vi "DT3120_GetFrameSize.vi"(8 "error in (no error)":errorcluster, 10 "Source":u16, 11 "DevId":i32) -> (0 "error out":errorcluster, 2 "Frame Size":T1, 3 "DevId (dup)":i32)   [LabVIEW 2013]
uses:
  olfg32.dll
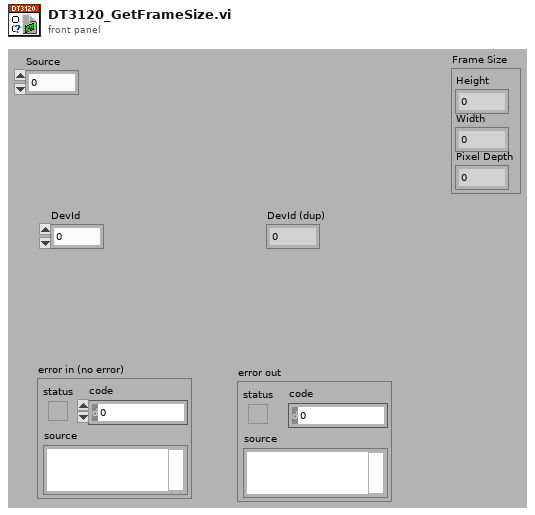
[diagram p1: front panel]
types:
  T1 = cluster{"Height":u32, "Width":u32, "Pixel Depth":u32}
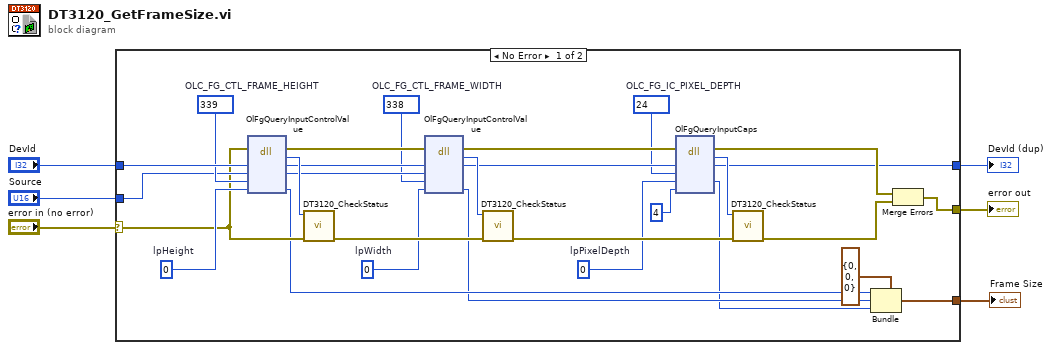
[diagram p0: block diagram]
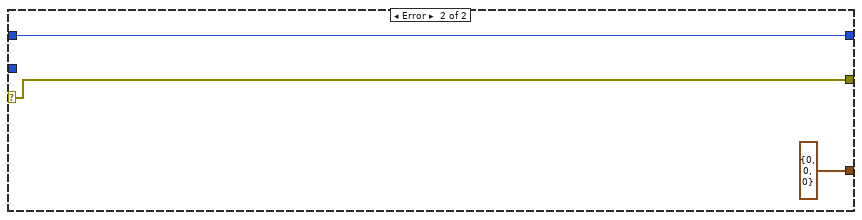
[diagram p2: hidden frame]
diagram:
  n1 = case shown="No Error" "error in (no error)" {
    selector: "error in (no error)" -> [w16 w38]
    tunnel: "DevId" -> [w34 w37]
    tunnel: "Source" -> [w27 _]
    tunnel: [w18 w38] -> w4
    tunnel: [w17 w37] -> w3
    tunnel: [w8 T1 {"Height"=0, "Width"=0, "Pixel Depth"=0} ("Frame Size")] -> w1
    frame No Error {
      w12 = u32 0  # lpPixelDepth
      w14 = 24  # OLC_FG_IC_PIXEL_DEPTH
      w15 = 338  # OLC_FG_CTL_FRAME_WIDTH
      w28 = u32 0  # lpWidth
      w32 = u32 0  # lpHeight
      w33 = 339  # OLC_FG_CTL_FRAME_HEIGHT
      n2 = dll-call lib="C:/Users/dhaehnel/Documents/Workspace/Labview_Workspace/labviewlib/MT Scan/SubVIs/olfg32.dll" fn="OlFgQueryInputControlValue"(error in=w16, "DevId"=w34, "Source"=w27, "Key"=w33, "lpValue"=w32) -> (error out=w31:errorcluster, "Status"=w35:u32, "DevId"=w25:i32, "Source"=w26:u16, "lpValue"=w11:u32)  [unwired: 3 in, 1 out]
      n3 = call "DT3120_CheckStatus.vi"("error in"=w16, "Status"=w35) -> ("error out"=w30:errorcluster)  [unwired: 9 out]
      n4 = dll-call lib="C:/Users/dhaehnel/Documents/Workspace/Labview_Workspace/labviewlib/MT Scan/SubVIs/olfg32.dll" fn="OlFgQueryInputControlValue"(error in=w31, "DevId"=w25, "Source"=w26, "Key"=w15, "lpValue"=w28) -> (error out=w23:errorcluster, "Status"=w29:u32, "DevId"=w24:i32, "lpValue"=w10:u32)  [unwired: 4 in, 1 out]
      n5 = call "DT3120_CheckStatus.vi"("error in"=w30, "Status"=w29) -> ("error out"=w21:errorcluster)  [unwired: 9 out]
      n6 = dll-call lib="C:/Users/dhaehnel/Documents/Workspace/Labview_Workspace/labviewlib/MT Scan/SubVIs/olfg32.dll" fn="OlFgQueryInputCaps"(error in=w23, "DevId"=w24, "Key"=w14, "lpData"=w12, "DataSize"=u32 4) -> (error out=w20:errorcluster, "Status"=w22:u32, "DevId"=w17:i32, "lpData"=w9:u32)  [unwired: 4 in, 1 out]
      n7 = call "DT3120_CheckStatus.vi"("error in"=w21, "Status"=w22) -> ("error out"=w19:errorcluster)  [unwired: 9 out]
      n8 = Bundle(cluster=T1 {"Height"=0, "Width"=0, "Pixel Depth"=0} ("Frame Size"), "Height"=w11, "Width"=w10, "Pixel Depth"=w9) -> (w8:T1)
      n9 = Merge Errors(w20, w19) -> (w18:errorcluster)
    }
    frame Error {
    }
  }
  "error out" <- w4
  "DevId (dup)" <- w3
  "Frame Size" <- w1
